vi "Test - Draw Line v2.vi"() -> ()   [LabVIEW 2022 SP3, in "Raster.lvlib"]
uses:
  Point 2D (I32).ctl
  Rectangle Dimensions.ctl
  Utility/Convert Pixels To Picture.vi/d601d993-a776-4dc8-89c7-357d8398c88c.vi
  Utility/Convert Pixels To Picture.vi/7816d0d6-8e4d-41a2-85ac-ed82f1435763.vi
  <vilib>/Utility/High Resolution Relative Seconds.vi
  <vilib>/picture/picture.llb/Draw Unflattened Pixmap.vi
  <vilib>/picture/picture.llb/Draw True-Color Pixmap.vi
  Raster.lvlib
  Utility/Utility.lvlib
panel:
  out "new picture":picture
  out "Pixel Data out":u32[][](array[colorbox])
  # "(0,0)"
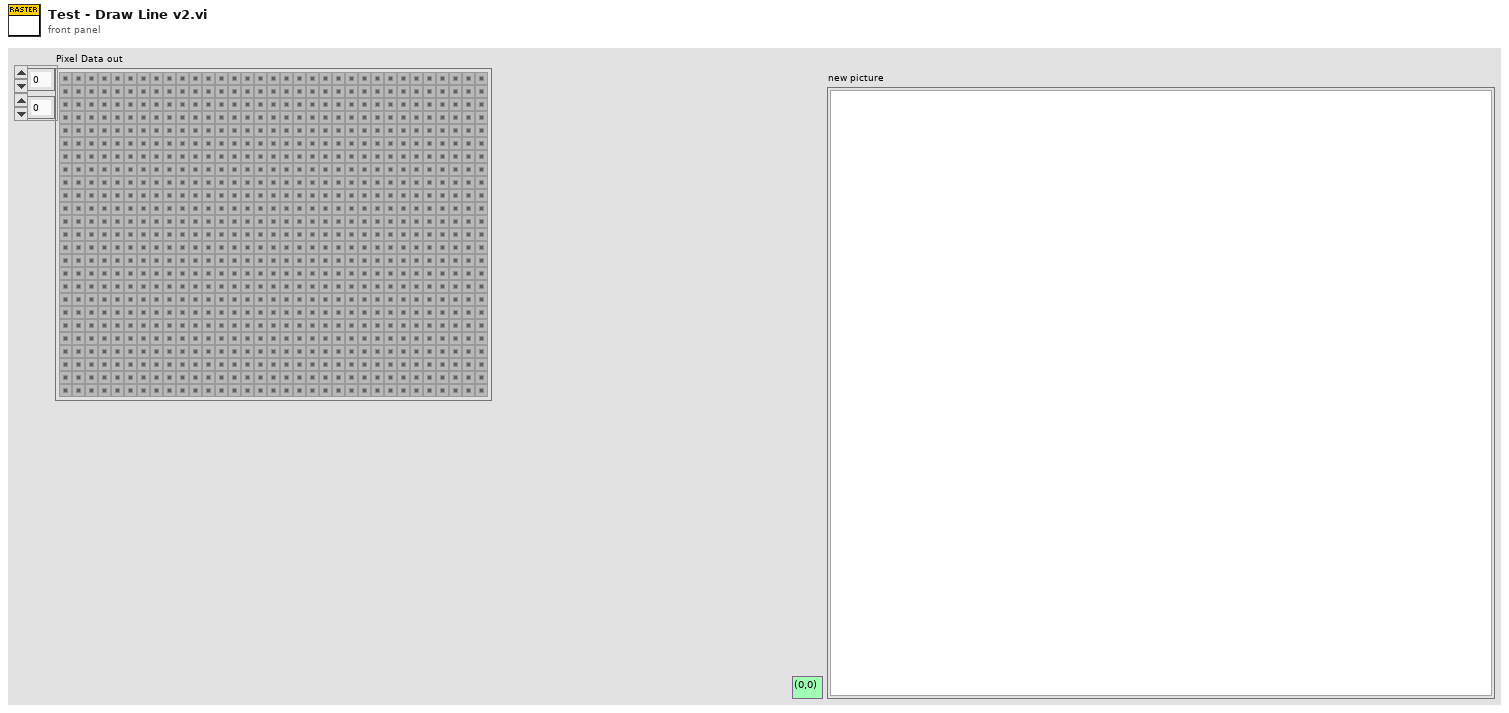
[diagram p1: front panel]
types:
  T1 = typedef "Raster.lvlib/Rectangle Dimensions.ctl" = cluster{"Width":u32, "Height":u32}
  T2 = typedef "Raster.lvlib/Point 2D (I32).ctl" = cluster{"x":i32, "y":i32}
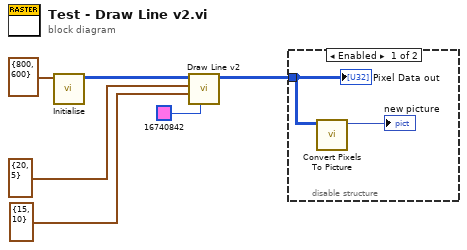
[diagram p0: block diagram]
diagram:
  n1 = call "Initialise.vi"("Screen Dimensions"=T1 {"Width"=800, "Height"=600}) -> ("Pixel Data out"=w6:u32[][])  [unwired: 10 in]
  n2 = call "Draw Line v2.vi"("Colour"=u32 16740842, "Point 2"=T2 {"x"=15, "y"=10} ("Point 1"), "Point 1"=T2 {"x"=20, "y"=5}, "Pixel Data in"=w6) -> ("Pixel Data out"=w3:u32[][])  [unwired: 7 in]
  n3 = disable-structure shown="Enabled" {
    disable-tunnel: w3 -> [w8 _]
    frame Enabled {
      n4 = call "Convert Pixels To Picture.vi"("Pixel Data in"=w8) -> ("2D Picture"=→"new picture":picture)  [unwired: 9 in, 1 out]
      "Pixel Data out" <- w8
    }
    frame Disabled {
    }
  }
